vi "Auto Piston.vi"(8 "error in (no error)":errorcluster, 11 "T=Forward, F=Reverse":bool) -> (0 "error out":errorcluster)   [LabVIEW 2014]
uses:
  <vilib>/Rock Robotics/WPI/Solenoid/WPI_SolenoidValue.ctl
  Global Variables/Global Variables.vi
  <vilib>/Rock Robotics/WPI/Solenoid/WPI_SolenoidSetEnum.vi
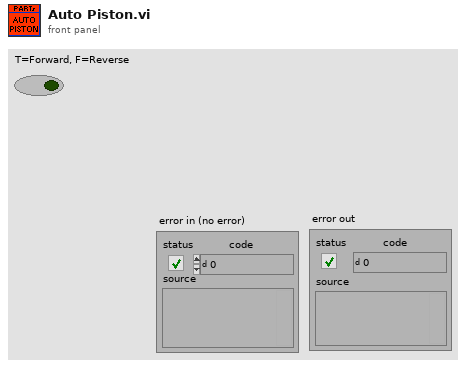
[diagram p1: front panel]
types:
  T1 = typedef "WPI_SolenoidValue.ctl" = enum16{"Off", "On", "Forward", "Reverse"}
  T2 = typedef "WPI_SolenoidDevRef.ctl" = cluster{"DevStatus":errorcluster, "Pneumatics Control Module":u8, "Forward Solenoid Channel":T3, "Reverse Solenoid Channel":T3}
  T3 = typedef "WPI_SolenoidChannel.ctl" = enum8{"Solenoid 0", "Solenoid 1", "Solenoid 2", "Solenoid 3", "Solenoid 4", "Solenoid 5", "Solenoid 6", "Solenoid 7", "Invalid"}
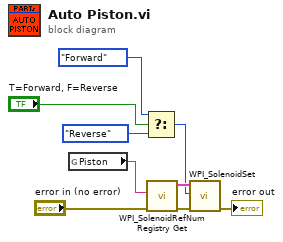
[diagram p0: block diagram]
diagram:
  n1 = global read "Global Variables.vi" "Piston"() -> (w4:string)
  n2 = Select(t=WPI_SolenoidValue."Forward" ("Value"), s="T=Forward, F=Reverse", f=WPI_SolenoidValue."Reverse" ("Value")) -> (s? t:f=w5:T1)
  n3 = call <vilib>:"WPI_SolenoidRefNum Registry Get.vi"("error in (no error)"="error in (no error)", "refnum name"=w4) -> ("error out"=w9:errorcluster, "SolenoidDevRef"=w8:T2)  [unwired: 8 in]
  n4 = call-poly <vilib>:"WPI_SolenoidSet.vi"("error in (no error)"=w9, "Value"=w5, "SolenoidDevRef"=w8) -> ("error out"=→"error out":errorcluster)  [unwired: 7 in, 1 out]
